vi "Read Data.vi"(8 "error in (no error)":errorcluster, 11 "Readable in":refnum<class "Readable.lvclass">) -> (0 "error out":errorcluster, 1 "Channel Names":string[](array[string]), 2 "Data Points":T4, 3 "Readable out":refnum<class "Readable.lvclass">, 4 "Channel Units":string[](array[string]), 5 "Data Channels":T1, 7 "#Channels":i32)   [LabVIEW 2009, in "Readable.lvclass"]
doc: "Perform a measurement and return one or more channels of data. Public interface to \"_Read.vi.\" (Use this one!)"
uses:
  Readable.lvclass
  Data Points.ctl
  Data Point.ctl
  Data Channel.ctl
  Data Channels.ctl
panel:
  in  "Data Channels constant":T2
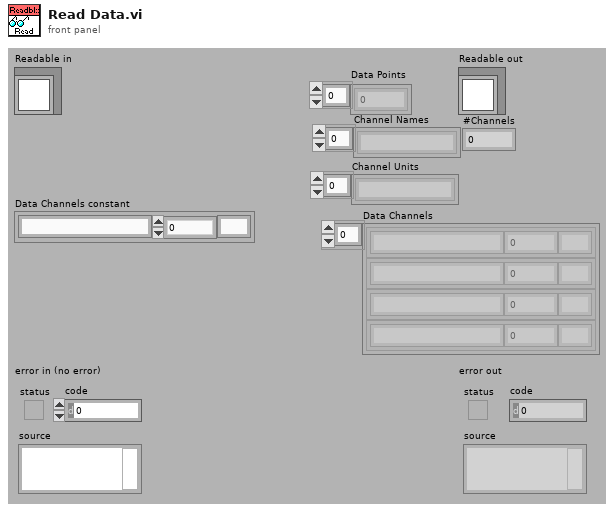
[diagram p1: front panel]
types:
  T1 = typedef "Readable.lvclass/Data Channels.ctl" = T2[]
  T2 = typedef "Readable.lvclass/Data Channel.ctl" = cluster{"Name":string, "Data Point":T3, "Unit":string}
  T3 = typedef "Readable.lvclass/Data Point.ctl" = dbl
  T4 = typedef "Readable.lvclass/Data Points.ctl" = T3[]
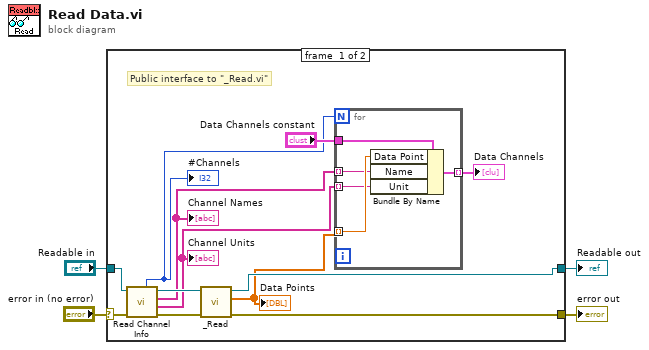
[diagram p0: block diagram]
diagram:
  n1 = case shown="No Error" "error in (no error)" {
    selector: "error in (no error)" -> [w12 w23]
    tunnel: [w16 w23] -> w3
    tunnel: [w14 w22] -> w1
    tunnel: "Readable in" -> [w15 w22]
    frame #0 {
      # "Public interface to \"_Read.vi\""
      n2 = call-dynamic "Read Channel Info.vi"("error in (no error)"=w12, "Readable.lvclass in"=w15) -> ("error out"=w11:errorcluster, "Channel Units"=w10:string[], "Channel Names"=w9:string[], "Readable.lvclass out"=w13:refnum<class "Readable.lvclass">, "#Channels"=w5:i32)  [unwired: 5 out]
      "#Channels" <- w5
      "Channel Names" <- w9
      "Channel Units" <- w10
      n3 = call-dynamic "_Read.vi"("error in (no error)"=w11, "Readable in"=w13) -> ("error out"=w16:errorcluster, "Data Points"=w8:T4, "Readable out"=w14:refnum<class "Readable.lvclass">)  [unwired: 7 out]
      "Data Points" <- w8
      n4 = for {
        N: w5 -> [_]
        tunnel: w8 -> [w21] mode=indexing
        tunnel: w9 -> [w19] mode=indexing
        tunnel: w10 -> [w18] mode=indexing
        tunnel: "Data Channels constant" -> [w20]
        tunnel: [w17] -> w6 mode=indexing
        n5 = Bundle By Name(cluster=w20, "Data Point"=w21, "Name"=w19, "Unit"=w18) -> (w17:T2)
      }
      "Data Channels" <- w6
    }
    frame #1 {
    }
  }
  "error out" <- w3
  "Readable out" <- w1
